vi "Emulator_Array.vi"() -> ()   [LabVIEW 2014]
panel:
  out "appended array 3":i64[](array[numeric])
  out "appended array 2":bool[](array[boolean])
  out "appended array":dbl[](array[numeric])
  in  "stop":bool
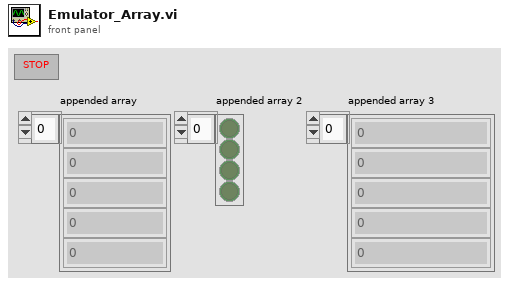
[diagram p1: front panel]
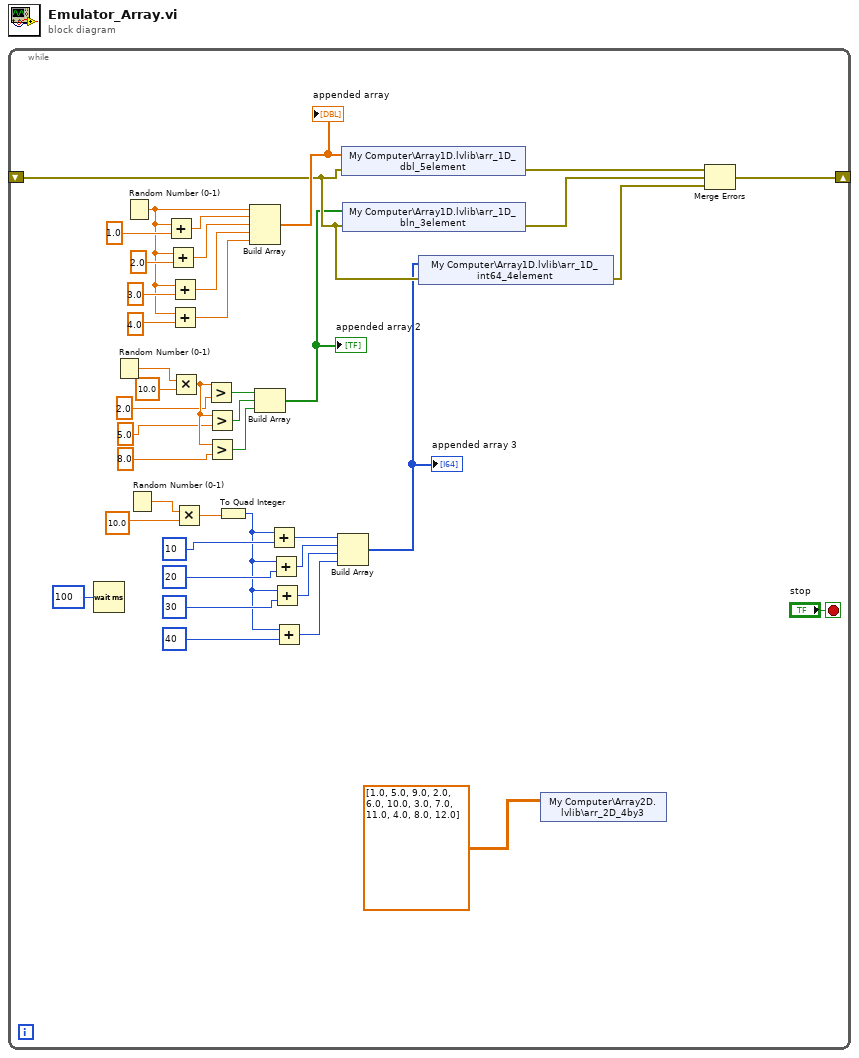
[diagram p0: block diagram]
diagram:
  n1 = while {
    shift-right: [w28] -> _
    shift-left: _ -> [w4]
    stop <- "stop" stop-if-true
    n2 = Wait (ms)(milliseconds to wait=u32 100) -> ()  [unwired: 1 out]
    n3 = Random Number (0-1)() -> (number: 0 to 1=w27:dbl)
    n4 = Random Number (0-1)() -> (number: 0 to 1=w33:dbl)
    n5 = Random Number (0-1)() -> (number: 0 to 1=w16:dbl)
    n6 = Add(x=w33, y=1.0) -> (x+y=w39:dbl)
    n7 = Add(x=w33, y=2.0) -> (x+y=w35:dbl)
    n8 = Add(x=w33, y=3.0) -> (x+y=w34:dbl)
    n9 = Add(x=w33, y=4.0) -> (x+y=w31:dbl)
    n10 = Multiply(x=w27, y=10.0) -> (x*y=w26:dbl)
    n11 = Multiply(x=w16, y=10.0) -> (x*y=w14:dbl)
    n12 = Greater?(x=w26, y=2.0) -> (0:w21:bool)
    n13 = Greater?(x=w26, y=5.0) -> (0:w20:bool)
    n14 = Greater?(x=w26, y=8.0) -> (0:w19:bool)
    n15 = To Quad Integer(1:w14) -> (0:w10:i64)
    n16 = Build Array(w33, w39, w35, w34, w31) -> (w30:dbl[])
    "appended array" <- w30
    n17 = Build Array(w21, w20, w19) -> (w2:bool[])
    "appended array 2" <- w2
    n18 = Add(x=w10, y=i64 10) -> (x+y=w8:i64)
    n19 = Add(x=w10, y=i64 20) -> (x+y=w7:i64)
    n20 = Add(x=w10, y=i64 30) -> (x+y=w6:i64)
    n21 = Add(x=w10, y=i64 40) -> (x+y=w5:i64)
    n22 = Build Array(w8, w7, w6, w5) -> (w3:i64[])
    "appended array 3" <- w3
    n23 = shared-variable "My Computer\\Array1D.lvlib\\arr_1D_dbl_5element"(w30, error in=w4) -> (error out=w29:errorcluster)
    n24 = shared-variable "My Computer\\Array1D.lvlib\\arr_1D_bln_3element"(w2, error in=w4) -> (error out=w18:errorcluster)
    n25 = shared-variable "My Computer\\Array1D.lvlib\\arr_1D_int64_4element"(w3, error in=w4) -> (error out=w17:errorcluster)
    n26 = shared-variable "My Computer\\Array2D.lvlib\\arr_2D_4by3"(dbl[][] [[1.0, 5.0, 9.0], [2.0, 6.0, 10.0], [3.0, 7.0, 11.0], [4.0, 8.0, 12.0]] ("arr_2D_4by3")) -> ()  [unwired: 1 in, 1 out]
    n27 = Merge Errors(w29, w18, w17) -> (w28:errorcluster)
  }
